vi "ReadBuffer.vi"(8 "error in (no error)":errorcluster, 9 "Combo Box":string(combo)="read", 10 "ServerConfig":string, 11 "Barcode":string) -> (0 "error out":errorcluster)   [LabVIEW 2024, in "FTPS.lvlib"]
doc: "This VI: Read Buffer \n------------------------------------------------\nreads the content of file giben in remote path \n------------------------------------------------\n-open the session with with FTP server using the credentials.\n-performs reads and write operation as per selection"
uses:
  FTPS.lvlib
  <vilib>/FTP/NI_FTP.lvlib
  Launcher/Launcher_DTU.lvlib
panel:
  in  "error in (no error) 2":errorcluster
  out "string array":string[][](array[string])
  out "delimited string":string
  in  "ClusterInputData":cluster{"Barcode":string, "ServerConfig":string}={"Barcode"="RRRTTT3", "ServerConfig"="SSLFile3"}
  in  "ClusterSetting":T1={"password"="1234", "user"="ftpadmin", "remote path"="/River/ssl_config.csv", "host"="169.254.73.100"}
  out "file error":errorcluster
  out "data":string
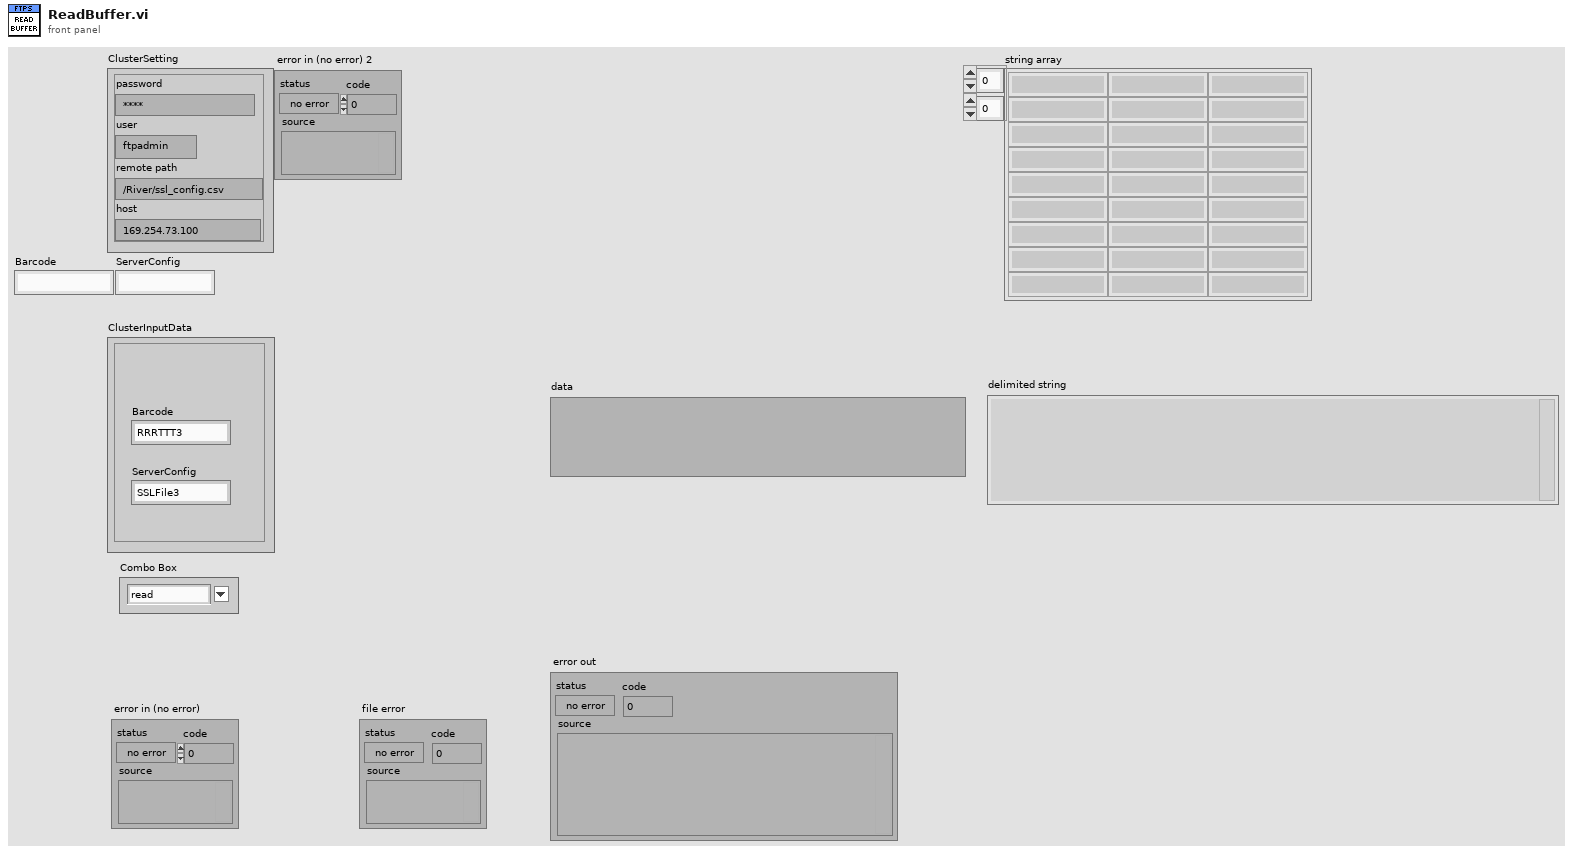
[diagram p1: front panel]
types:
  T1 = cluster{"password":string, "user":string, "remote path":string, "host":string}
  T2 = enum16{"Read", "Write", "All_sections", "All_values", "Remove key&section"}
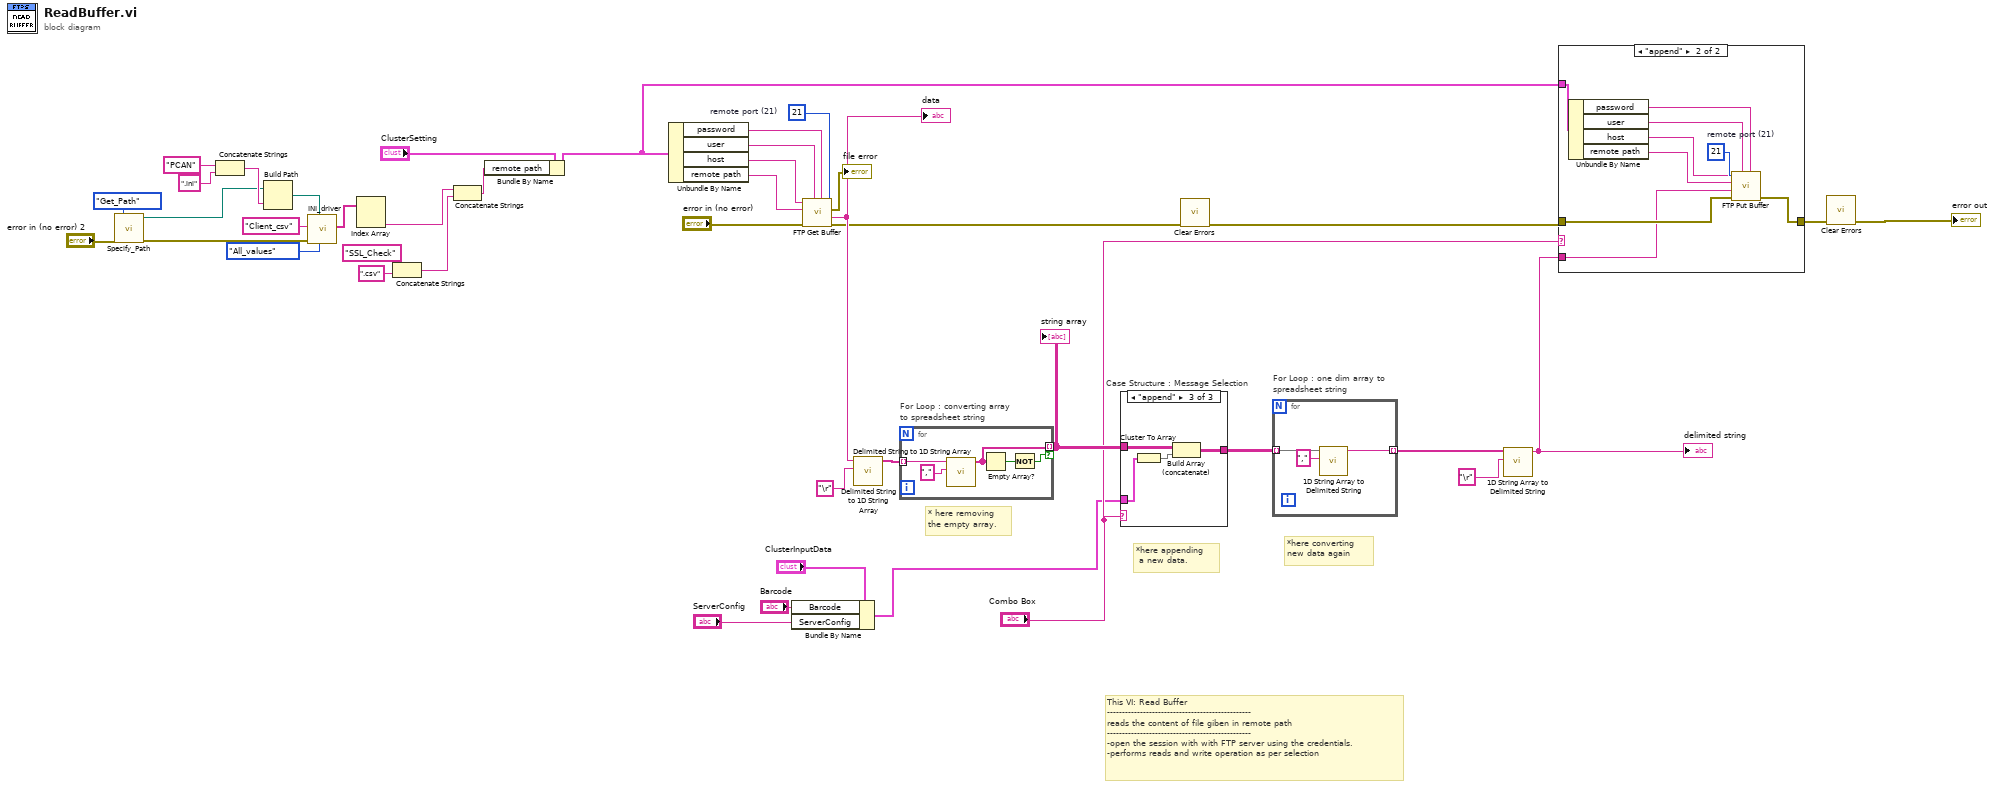
[diagram p0: block diagram]
diagram:
  w42 = u16 21  # remote port (21)
  # "*here converting \nnew data again"
  # "*here appending\n a new data."
  # "* here removing \nthe empty array."
  # "This VI: Read Buffer \n------------------------------------------------\nreads the content of file giben in remote path  \n------------------------------------------------\n-open the session with with FTP server using the credentials.\n-performs reads and write operation as per selection"
  n1 = call "Specify_Path.vi"("Path_Enum"=enum16{"Find_Path", "Get_Path"}."Get_Path", "error in (no error)"="error in (no error) 2") -> ("Configurations"=w11:path, "error out"=w15:errorcluster)  [unwired: 6 in, 6 out]
  n2 = Concatenate Strings("PCAN" ("string"), ".ini" ("string")) -> (w17:string)
  n3 = Build Path(base path=w11, name or relative path=w17) -> (appended path=w16:path)
  n4 = call "INI_driver.vi"("Enum"=T2."All_values", "instrument file path"=w16, "error in (no error)"=w15, "Section"="Client_csv") -> ("Values out"=w9:string[])  [unwired: 4 in, 3 out]
  n5 = Index Array(array=w9) -> (element #2=w5:string)  [unwired: 2 in, 1 out]
  n6 = Concatenate Strings("SSL_Check" ("string"), ".csv" ("string")) -> (w4:string)
  n7 = Concatenate Strings(w5, w4) -> (w6:string)
  n8 = Bundle By Name(cluster="ClusterSetting", "remote path"=w6) -> (w7:T1)
  n9 = Unbundle By Name(w7) -> ("password"=w33:string, "user"=w34:string, "host"=w35:string, "remote path"=w32:string)
  n10 = Bundle By Name(cluster="ClusterInputData", "Barcode"="Barcode", "ServerConfig"="ServerConfig") -> (w22:cluster{"Barcode":string, "ServerConfig":string})
  n11 = call <vilib>:"FTP Get Buffer.vi"("remote port (21)"=w42, "password"=w33, "user"=w34, "error in (no error)"="error in (no error)", "remote path"=w32, "host"=w35) -> ("error out"=w27:errorcluster, "data"=w39:string, "file error"=→"file error":errorcluster)  [unwired: 3 in]
  "data" <- w39
  n12 = call <vilib>:"Delimited String to 1D String Array.vi"("delimiter"="\r", "delimited string"=w39) -> ("string array"=w37:string[])  [unwired: 9 in]
  n13 = for "For Loop : converting array \nto spreadsheet string" {
    tunnel: w37 -> [w47] mode=indexing
    tunnel: [w45] -> w36 mode=indexing if=w43
    n14 = call <vilib>:"Delimited String to 1D String Array.vi"("delimiter"=",", "delimited string"=w47) -> ("string array"=w45:string[])  [unwired: 9 in]
    n15 = Empty Array?(array=w45) -> (empty?=w44:bool)
    n16 = Not(x=w44) -> (.not. x?=w43:bool)
  }
  "string array" <- w36
  n17 = case "Case Structure : Message Selection" shown="\"append\"" "Combo Box" {
    tunnel: w36 -> [_ w48 w52]
    tunnel: [_ w48 w51] -> w31
    tunnel: w22 -> [_ _ w50]
    frame "idle", Default {
    }
    frame "read" {
    }
    frame "append" {
      n18 = Cluster To Array(cluster=w50) -> (array=w49:string[])
      n19 = Build Array (concatenate)(w52, w49) -> (w51:string[][])
    }
  }
  n20 = call <vilib>:"Clear Errors.vi"("error in (no error)"=w27) -> ("error out"=w3:errorcluster)  [unwired: 5 in, 1 out]
  n21 = for "For Loop : one dim array to \nspreadsheet string" {
    tunnel: w31 -> [w55] mode=indexing
    tunnel: [w53] -> w30 mode=indexing
    n22 = call <vilib>:"1D String Array to Delimited String.vi"("delimiter"=",", "string array"=w55) -> ("delimited string"=w53:string)  [unwired: 9 in]
  }
  n23 = call <vilib>:"1D String Array to Delimited String.vi"("delimiter"="\r", "string array"=w30) -> ("delimited string"=w25:string)  [unwired: 9 in]
  "delimited string" <- w25
  n24 = case shown="\"append\"" "Combo Box" {
    tunnel: w7 -> [_ w65]
    tunnel: w3 -> [w56 w59]
    tunnel: [w56 w58] -> w26
    tunnel: w25 -> [_ w57]
    frame "False", Default {
    }
    frame "append" {
      w64 = u16 21  # remote port (21)
      n25 = Unbundle By Name(w65) -> ("password"=w63:string, "user"=w62:string, "host"=w61:string, "remote path"=w60:string)
      n26 = call <vilib>:"FTP Put Buffer.vi"("remote port (21)"=w64, "password"=w63, "user"=w62, "error in (no error)"=w59, "data"=w57, "remote path"=w60, "host"=w61) -> ("error out"=w58:errorcluster)  [unwired: 3 in, 1 out]
    }
  }
  n27 = call <vilib>:"Clear Errors.vi"("error in (no error)"=w26) -> ("error out"=→"error out":errorcluster)  [unwired: 5 in, 1 out]
